vi "FGV Map DeInit.vi"(8 "error in":errorcluster) -> (0 "error out":errorcluster)   [LabVIEW 2020, in "FGV Map.lvlib"]
uses:
  FGV Map.lvlib
  Controls/FGV Map Core State.ctl
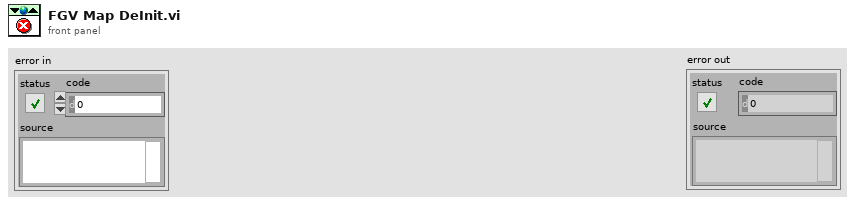
[diagram p1: front panel]
types:
  T1 = typedef "FGV Map.lvlib/FGV Map Core State.ctl" = enum16{"Init", "Set Instance (Unlock)", "Get Instance", "Get Instance (Lock)", "Unlock", "Get All Instances", "Delete Instance"}
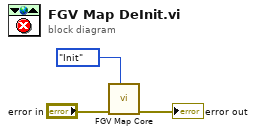
[diagram p0: block diagram]
diagram:
  n1 = call "FGV Map Core.vi"("FGV State"=FGV_Map_Core_State."Init", "error in"="error in") -> ("error out"=→"error out":errorcluster)  [unwired: 5 in, 4 out]
